vi "Set.vi"(0 "VISA resource name":refnum<visa-resource-name>, 1 "Local Lockout (0:1)":u32(ring) items=["Off", "On"], 2 "ATTN (0:1)":u32(ring) items=["Off", "On"], 3 "Run/Stop (1:0)":u32(ring)=1 items=["Stop", "Run"], 5 "Wavelength (nnnn)":dbl[unit]=8.210000000000001e-07, 6 "AVG (1:3)":u32(ring)=2 items=["Slow"=1, "Medium"=2, "Fast"=3], 9 "Range (0-Auto,1:8)":u32(ring) items=["Auto", "Lowest", "2", "3", "4", "5", "6", "7", "Highest"], 10 "Units (1:4)":u32(ring)=1 items=["W"=1, "dB"=2, "dBm"=3, "REL"=4], 11 "error in (no error)":errorcluster, 12 "Backlight (0:2)":u32(ring)=1 items=["Off", "Low", "High"], 13 "Beeper (0:1)":u32(ring) items=["Off", "On"], 14 "Zero (0:1)":u32(ring) items=["Off", "On"]) -> (4 "VISA resource name out":refnum<visa-resource-name>, 15 "error out":errorcluster)   [LabVIEW 2013]
doc: "Sets 1830-C options in succession."
uses:
  <vilib>/Utility/error.llb/DialogType.ctl
  Newport 1830-C.lvlib
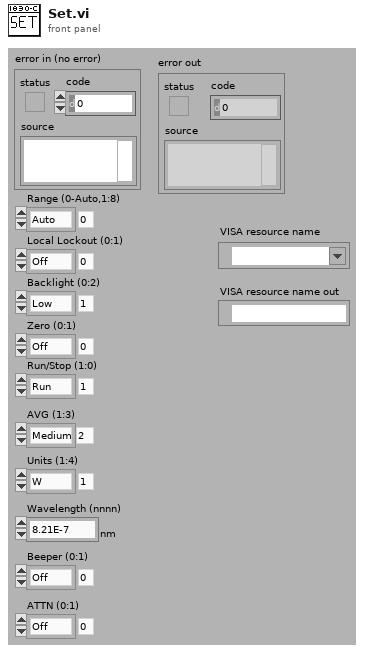
[diagram p1: front panel]
types:
  T1 = typedef "DialogType.ctl" = u16
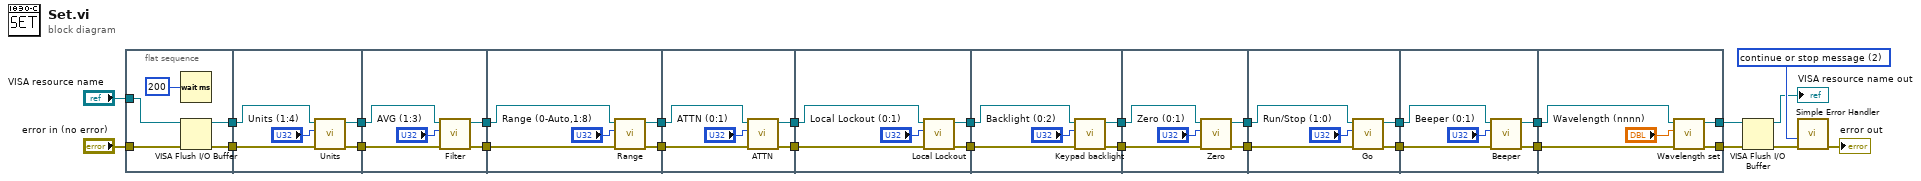
[diagram p0: block diagram]
diagram:
  w6 = T1 2 items=["no dialog", "OK message", "continue or stop message", "OK message + warnings", "continue/stop + warnings"] ("type of dialog (OK msg:1)")
  n1 = flat-sequence {
    tunnel: "error in (no error)" -> [w30]
    tunnel: "VISA resource name" -> [w29]
    tunnel: [w31] -> w8
    tunnel: [w32] -> w5
    tunnel: [w36] -> w27
    tunnel: [w34] -> w17
    tunnel: w8 -> [w35]
    tunnel: w5 -> [w37]
    tunnel: w27 -> [w42]
    tunnel: [w41] -> w25
    tunnel: w17 -> [w40]
    tunnel: [w39] -> w16
    tunnel: w25 -> [w47]
    tunnel: [w46] -> w24
    tunnel: w16 -> [w45]
    tunnel: [w44] -> w15
    tunnel: w24 -> [w52]
    tunnel: [w51] -> w23
    tunnel: w15 -> [w50]
    tunnel: [w49] -> w14
    tunnel: w23 -> [w57]
    tunnel: [w56] -> w22
    tunnel: w14 -> [w55]
    tunnel: [w54] -> w13
    tunnel: w22 -> [w62]
    tunnel: [w61] -> w21
    tunnel: w13 -> [w60]
    tunnel: [w59] -> w12
    tunnel: w21 -> [w67]
    tunnel: [w66] -> w20
    tunnel: w12 -> [w65]
    tunnel: [w64] -> w11
    tunnel: w20 -> [w72]
    tunnel: [w71] -> w19
    tunnel: w11 -> [w70]
    tunnel: [w69] -> w10
    tunnel: w19 -> [w77]
    tunnel: [w76] -> w18
    tunnel: w10 -> [w75]
    tunnel: [w74] -> w9
    tunnel: w18 -> [w82]
    tunnel: [w81] -> w2
    tunnel: [w80] -> w4
    tunnel: w9 -> [w79]
    frame #0 {
      n2 = Wait (ms)(milliseconds to wait=u32 200) -> ()  [unwired: 1 out]
      n3 = VISA Flush I/O Buffer(VISA resource name=w29, error in (no error)=w30) -> (VISA resource name out=w32:refnum<visa-resource-name>, error out=w31:errorcluster)  [unwired: 1 in]
    }
    frame #1 {
      n4 = call "Units.vi"("error in (no error)"=w35, "Units"="Units (1:4)", "VISA resource name"=w37) -> ("error out"=w34:errorcluster, "VISA resource name out"=w36:refnum<visa-resource-name>)  [unwired: 7 in]
    }
    frame #2 {
      n5 = call "Filter.vi"("error in (no error)"=w40, "Filter"="AVG (1:3)", "VISA resource name"=w42) -> ("error out"=w39:errorcluster, "VISA resource name out"=w41:refnum<visa-resource-name>)  [unwired: 7 in]
    }
    frame #3 {
      n6 = call "Range.vi"("error in (no error)"=w45, "Range"="Range (0-Auto,1:8)", "VISA resource name"=w47) -> ("error out"=w44:errorcluster, "VISA resource name out"=w46:refnum<visa-resource-name>)  [unwired: 7 in]
    }
    frame #4 {
      n7 = call "ATTN.vi"("error in (no error)"=w50, "Attn"="ATTN (0:1)", "VISA resource name"=w52) -> ("error out"=w49:errorcluster, "VISA resource name out"=w51:refnum<visa-resource-name>)  [unwired: 7 in]
    }
    frame #5 {
      n8 = call "Local Lockout.vi"("error in (no error)"=w55, "Local Lockout"="Local Lockout (0:1)", "VISA resource name"=w57) -> ("error out"=w54:errorcluster, "VISA resource name out"=w56:refnum<visa-resource-name>)  [unwired: 7 in]
    }
    frame #6 {
      n9 = call "Keypad backlight.vi"("error in (no error)"=w60, "BKLT"="Backlight (0:2)", "VISA resource name"=w62) -> ("error out"=w59:errorcluster, "VISA resource name out"=w61:refnum<visa-resource-name>)  [unwired: 7 in]
    }
    frame #7 {
      n10 = call "Zero.vi"("error in (no error)"=w65, "Zero"="Zero (0:1)", "VISA resource name"=w67) -> ("error out"=w64:errorcluster, "VISA resource name out"=w66:refnum<visa-resource-name>)  [unwired: 7 in]
    }
    frame #8 {
      n11 = call "Go.vi"("error in (no error)"=w70, "Run/Stop"="Run/Stop (1:0)", "VISA resource name"=w72) -> ("error out"=w69:errorcluster, "VISA resource name out"=w71:refnum<visa-resource-name>)  [unwired: 7 in]
    }
    frame #9 {
      n12 = call "Beeper.vi"("error in (no error)"=w75, "Beeper"="Beeper (0:1)", "VISA resource name"=w77) -> ("error out"=w74:errorcluster, "VISA resource name out"=w76:refnum<visa-resource-name>)  [unwired: 7 in]
    }
    frame #10 {
      n13 = call "Wavelength set.vi"("error in (no error)"=w79, "Wavelength (nnnn)"="Wavelength (nnnn)", "VISA resource name"=w82) -> ("error out"=w80:errorcluster, "VISA resource name out"=w81:refnum<visa-resource-name>)  [unwired: 7 in]
    }
  }
  n14 = VISA Flush I/O Buffer(VISA resource name=w2, error in (no error)=w4) -> (VISA resource name out=→"VISA resource name out":refnum<visa-resource-name>, error out=w3:errorcluster)  [unwired: 1 in]
  n15 = call <vilib>:"Simple Error Handler.vi"("type of dialog (OK msg:1)"=w6, "error in (no error)"=w3) -> ("error out"=→"error out":errorcluster)  [unwired: 3 in, 4 out]
